vi "remove lvclass extension.vi"(11 "class name in":string) -> (3 "class name out":string)   [LabVIEW 2013, in "NISE_CEF_class discovery library.lvlib"]
doc: "Removes the .lvclass extension from a string. Foo.lvclass becomes foo. Blah.lvlib::foo.lvclass becomes Blah.lvlib::foo"
uses:
  NISE_CEF_class discovery library.lvlib
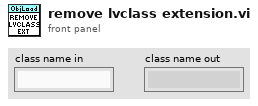
[diagram p1: front panel]
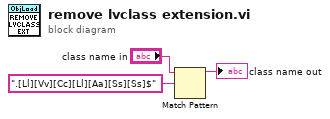
[diagram p0: block diagram]
diagram:
  n1 = Match Pattern(string="class name in", regular expression=".[Ll][Vv][Cc][Ll][Aa][Ss][Ss]$") -> (before substring=→"class name out":string)  [unwired: 1 in, 3 out]
